vi "configure_udc.vi"() -> ()   [LabVIEW 2011]
panel:
  in  "Write":bool
  in  "Read":bool
  out "Value Array":dbl[](array[numeric])
  out "Transfer Bar":u8(slide) caption="Transfer progress..." scale=0.0..100.0
  out "Current Value":dbl caption="Current Value:"
  in  "New Value":dbl caption="New Value:"
  in  "Upload Values":bool
  in  "Download Values":bool
  in  "Load Configuration":bool
  in  "Save Configuration":bool
  in  "Exit":bool
  in  "Parameters":i32(listbox)
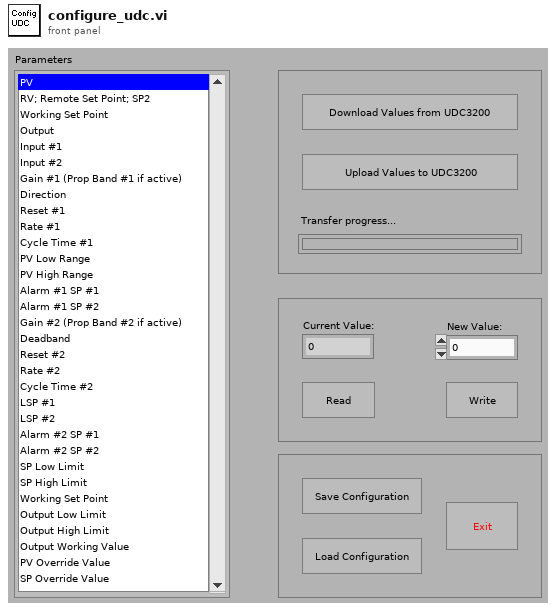
[diagram p1: front panel]
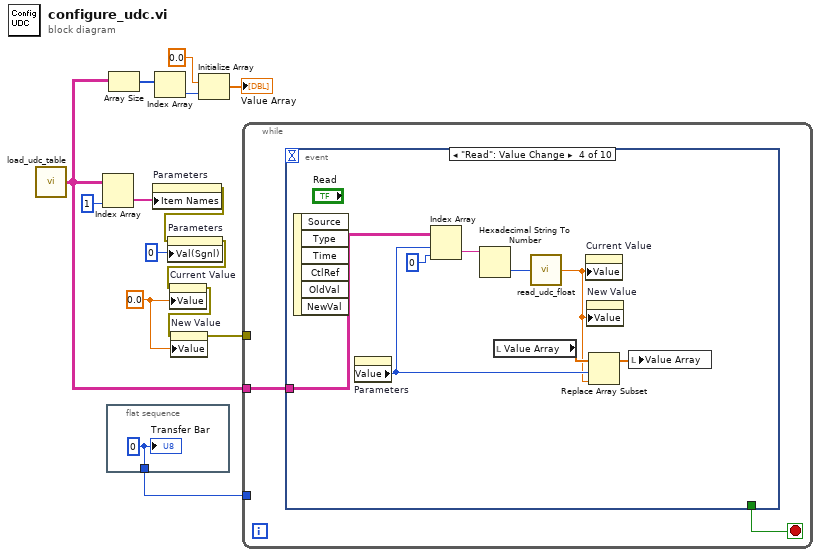
[diagram p0: block diagram]
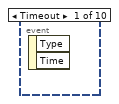
[diagram p2: hidden frame]
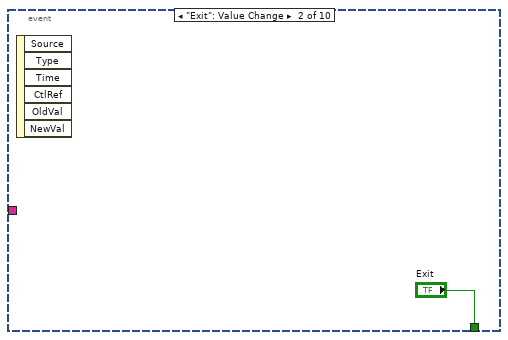
[diagram p3: hidden frame]
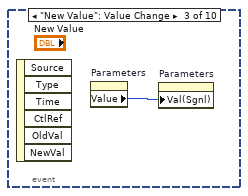
[diagram p4: hidden frame]
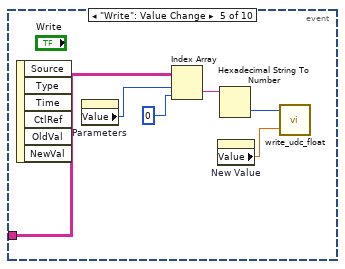
[diagram p5: hidden frame]
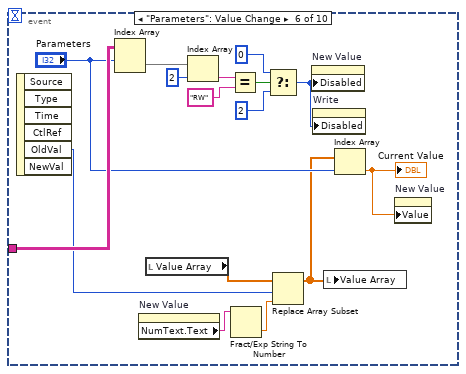
[diagram p6: hidden frame]
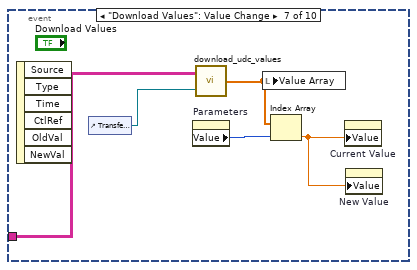
[diagram p7: hidden frame]
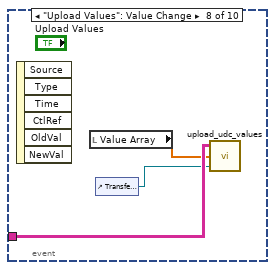
[diagram p8: hidden frame]
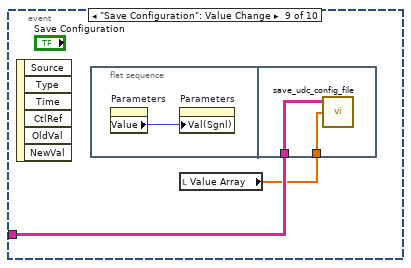
[diagram p9: hidden frame]
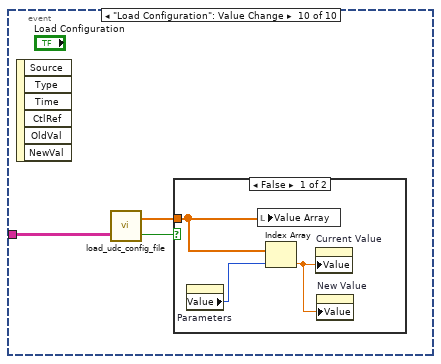
[diagram p10: hidden frame]
diagram:
  w5 = 0.0 ("Current Value")
  n1 = call "load_udc_table.vi"() -> ("UDC Table"=w10:string[][])  [unwired: 1 out]
  n2 = Index Array(array=w10, index (col)=1 ("disabled index (col)")) -> (element=w13:string[])  [unwired: 1 in]
  n3 = flat-sequence {
    tunnel: [w15] -> w2
    frame #0 {
      w15 = u8 0 ("Transfer in progress...")
      "Transfer Bar" <- w15
    }
  }
  n4 = Array Size(array=w10) -> (size(s)=w9:i32[])
  n5 = property on="Parameters" class="LstBox (strict)"("Item Names"=w13) -> (error out=w11:errorcluster)  [unwired: 2 in, 1 out]
  n6 = Index Array(array=w9) -> (element=w8:i32)  [unwired: 1 in]
  n7 = property on="Parameters" class="LstBox (strict)"(error in=w11, "Val(Sgnl)"=0 ("Parameters")) -> (error out=w3:errorcluster)  [unwired: 1 in, 1 out]
  n8 = property on="Current Value" class="DigNum (strict)"(error in=w3, "Value"=w5) -> (error out=w6:errorcluster)  [unwired: 1 in, 1 out]
  n9 = property on="New Value" class="DigNum (strict)"(error in=w6, "Value"=w5) -> (error out=w4:errorcluster)  [unwired: 1 in, 1 out]
  n10 = Initialize Array(0.0, w8) -> (→"Value Array":dbl[])
  n11 = while {
    tunnel: w10 -> [w16]
    tunnel: w4 -> [_]
    tunnel: w2 -> [_]
    stop <- w17 stop-if-true
    n12 = event shown="[3] \"Read\": Value Change" {
      selector: _ -> [_ _ _ _ _ _ _ _ _ _]
      dyn-events: _ -> [_ _ _ _ _ _ _ _ _ _]
      timeout: _ -> [_ _ _ _ _ _ _ _ _ _]
      tunnel: [_ "Exit" _ _ _ _ _ _ _ _] -> w17
      tunnel: w16 -> [_ _ _ w27 w33 w49 w54 w57 w59 w65]
      event Timeout {
        n13 = event-data() -> ()  [unwired: 3 out]
      }
      event "Exit": Value Change {
        n14 = event-data() -> ()  [unwired: 7 out]
      }
      event "New Value": Value Change {
        n15 = event-data() -> ()  [unwired: 7 out]
        n16 = property on="Parameters" class="LstBox (strict)"() -> ("Value"=w19:i32)  [unwired: 2 in, 2 out]
        n17 = property on="Parameters" class="LstBox (strict)"("Val(Sgnl)"=w19) -> ()  [unwired: 2 in, 2 out]
      }
      event "Read": Value Change {
        n18 = event-data() -> ()  [unwired: 7 out]
        n19 = property on="Parameters" class="LstBox (strict)"() -> ("Value"=w22:i32)  [unwired: 2 in, 2 out]
        n20 = Index Array(array=w27, index (row)=w22, index (col)=0 ("disabled index (col)")) -> (element=w25:string)
        n21 = Hexadecimal String To Number(string=w25) -> (number=w24:u32)  [unwired: 3 out]
        n22 = local read "Value Array"() -> (w23:dbl[])
        n23 = call "read_udc_float.vi"("Hex Address"=w24) -> ("Value"=w21:dbl)
        n24 = property on="Current Value" class="DigNum (strict)"("Value"=w21) -> ()  [unwired: 2 in, 2 out]
        n25 = property on="New Value" class="DigNum (strict)"("Value"=w21) -> ()  [unwired: 2 in, 2 out]
        n26 = Replace Array Subset(array=w23, new element=w21, index=w22) -> (w20:dbl[])
        n27 = local write "Value Array"(w20) -> ()
      }
      event "Write": Value Change {
        n28 = event-data() -> ()  [unwired: 7 out]
        n29 = property on="Parameters" class="LstBox (strict)"() -> ("Value"=w29:i32)  [unwired: 2 in, 2 out]
        n30 = Index Array(array=w33, index (row)=w29, index (col)=0 ("disabled index (col)")) -> (element=w31:string)
        n31 = property on="New Value" class="DigNum (strict)"() -> ("Value"=w28:dbl)  [unwired: 2 in, 2 out]
        n32 = Hexadecimal String To Number(string=w31) -> (number=w30:u32)  [unwired: 3 out]
        n33 = call "write_udc_float.vi"("Value"=w28, "Hex Address"=w30) -> ()  [unwired: 1 out]
      }
      event "Parameters": Value Change {
        n34 = event-data() -> ("OldVal"=w40:i32)  [unwired: 6 out]
        n35 = Index Array(array=w49, index (row)="Parameters") -> (element=w42:string[])  [unwired: 1 in]
        n36 = property on="New Value" class="DigNum (strict)"() -> ("NumText.Text"=w39:string)  [unwired: 2 in, 2 out]
        n37 = local read "Value Array"() -> (w36:dbl[])
        n38 = Index Array(array=w42, index=2) -> (element=w47:string)
        n39 = Equal?(x=w47, y="RW") -> (x = y?=w45:bool)
        n40 = Fract/Exp String To Number(string=w39) -> (number=w37:dbl)  [unwired: 4 out]
        n41 = Select(t=u8 0 ("Disabled"), s=w45, f=u8 2 ("Disabled")) -> (s? t:f=w34:u8)
        n42 = Replace Array Subset(array=w36, new element=w37, index=w40) -> (w35:dbl[])
        n43 = property on="New Value" class="DigNum (strict)"("Disabled"=w34) -> ()  [unwired: 2 in, 2 out]
        n44 = property on="Write" class="Bool"("Disabled"=w34) -> ()  [unwired: 2 in, 2 out]
        n45 = local write "Value Array"(w35) -> ()
        n46 = Index Array(array=w35, index="Parameters") -> (element=w38:dbl)
        "Current Value" <- w38
        n47 = property on="New Value" class="DigNum (strict)"("Value"=w38) -> ()  [unwired: 2 in, 2 out]
      }
      event "Download Values": Value Change {
        n48 = event-data() -> ()  [unwired: 7 out]
        n49 = control-ref of="Transfer Bar"() -> (w53:refnum<vi>)
        n50 = property on="Parameters" class="LstBox (strict)"() -> ("Value"=w51:i32)  [unwired: 2 in, 2 out]
        n51 = call "download_udc_values.vi"("Transfer Bar"=w53, "UDC Table"=w54) -> ("Value Array"=w52:dbl[])
        n52 = local write "Value Array"(w52) -> ()
        n53 = Index Array(array=w52, index=w51) -> (element=w50:dbl)
        n54 = property on="Current Value" class="DigNum (strict)"("Value"=w50) -> ()  [unwired: 2 in, 2 out]
        n55 = property on="New Value" class="DigNum (strict)"("Value"=w50) -> ()  [unwired: 2 in, 2 out]
      }
      event "Upload Values": Value Change {
        n56 = event-data() -> ()  [unwired: 7 out]
        n57 = local read "Value Array"() -> (w55:dbl[])
        n58 = control-ref of="Transfer Bar"() -> (w56:refnum<vi>)
        n59 = call "upload_udc_values.vi"("Transfer Bar"=w56, "Value Array"=w55, "UDC Table"=w57) -> ()  [unwired: 1 out]
      }
      event "Save Configuration": Value Change {
        n60 = event-data() -> ()  [unwired: 7 out]
        n61 = flat-sequence {
          tunnel: w59 -> [w62]
          tunnel: w58 -> [w61]
          frame #0 {
            n62 = property on="Parameters" class="LstBox (strict)"() -> ("Value"=w60:i32)  [unwired: 2 in, 2 out]
            n63 = property on="Parameters" class="LstBox (strict)"("Val(Sgnl)"=w60) -> ()  [unwired: 2 in, 2 out]
          }
          frame #1 {
            n64 = call "save_udc_config_file.vi"("Value Array"=w61, "UDC Table"=w62) -> ()  [unwired: 1 in, 1 out]
          }
        }
        n65 = local read "Value Array"() -> (w58:dbl[])
      }
      event "Load Configuration": Value Change {
        n66 = event-data() -> ()  [unwired: 7 out]
        n67 = call "load_udc_config_file.vi"("UDC Table"=w65) -> ("Cancelled"=w64:bool, "Array"=w63:dbl[])  [unwired: 1 in]
        n68 = case shown="False" w64 {
          tunnel: w63 -> [w68 _]
          frame False {
            n69 = property on="Parameters" class="LstBox (strict)"() -> ("Value"=w67:i32)  [unwired: 2 in, 2 out]
            n70 = local write "Value Array"(w68) -> ()
            n71 = Index Array(array=w68, index=w67) -> (element=w66:dbl)
            n72 = property on="Current Value" class="DigNum (strict)"("Value"=w66) -> ()  [unwired: 2 in, 2 out]
            n73 = property on="New Value" class="DigNum (strict)"("Value"=w66) -> ()  [unwired: 2 in, 2 out]
          }
          frame True {
          }
        }
      }
    }
  }
